vi "StreamDAQ.vi"(1 "Control refDes array":string[][](array[string]), 5 "Control Data Type":dbl[](array[numeric]), 7 "Logging Queue":refnum<queue>, 9 "StreamCluster_TypeDef":T1={"DAQ_Configs"=[], "CTR_Config"={"CTR refDes"="CTR001", "CTR IP Addr"="localhost", "Restart"=FALSE}, "Network_Configs"={"Buffer"=1, "ManagmentRate_Hz"=1000, "StreamRate_Hz"=10, "ConnectionHysterisis"=0, "LoggingRate_Hz"=10}, "ConfigXML_Checksum"=""}, 11 "error in":errorcluster) -> (6 "Control Data Out":dbl[](array[numeric]), 10 "StreamCluster_TypeDef":T1={"DAQ_Configs"=[], "CTR_Config"={"CTR refDes"="CTR001", "CTR IP Addr"="localhost", "Restart"=FALSE}, "Network_Configs"={"Buffer"=1, "ManagmentRate_Hz"=1000, "StreamRate_Hz"=10, "ConnectionHysterisis"=0, "LoggingRate_Hz"=10}, "ConfigXML_Checksum"=""}, 15 "error out":errorcluster)   [LabVIEW 2024]
uses:
  OneDrive - Embry-Riddle Aeronautical University/Admin/Facilities/TC3/TC3 DAC/Code/RTC_PXIe-Code v1_9_0 CODE/QMH-Architecture/support/Control/StreamCluster_TypeDef.ctl
  Control/streamIO_states.ctl
panel:
  out "timed out? 2":bool
  out "timed out?":bool
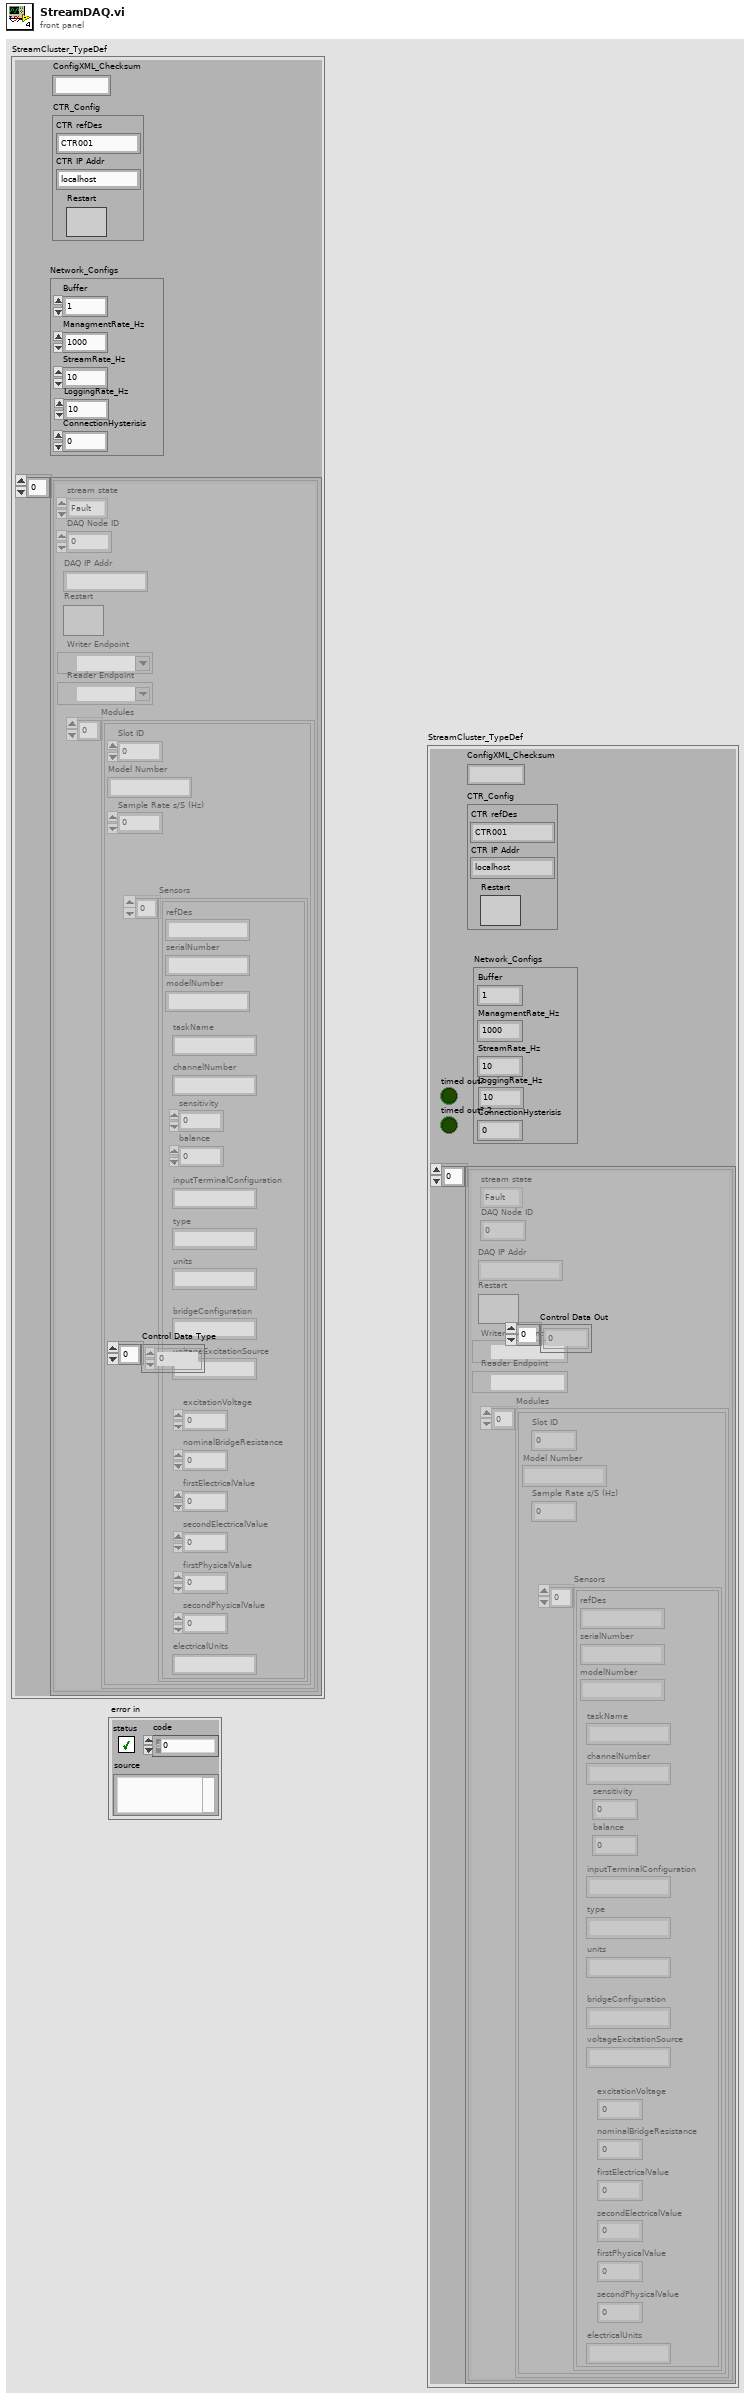
[diagram p1: front panel]
types:
  T1 = typedef "StreamCluster_TypeDef.ctl" = cluster{"DAQ_Configs":cluster{"stream state":T2, "DAQ Node ID":i32, "Writer Endpoint":refnum<k21>, "Reader Endpoint":refnum<k21>, "Modules":cluster{"Slot ID":i32, "Model Number":string, "Sample Rate s/S (Hz)":dbl, "Sensors":cluster{"refDes":string, "serialNumber":string, "modelNumber":string, "units":string, "balance":dbl, "sensitivity":dbl, "type":string, "inputTerminalConfiguration":string, "channelNumber":string, "taskName":string, "bridgeConfiguration":string, "excitationVoltage":dbl, "voltageExcitationSource":string, "nominalBridgeResistance":dbl, "firstElectricalValue":dbl, "secondElectricalValue":dbl, "firstPhysicalValue":dbl, "secondPhysicalValue":dbl, "electricalUnits":string}[]}[], "DAQ IP Addr":string, "Restart":bool}[], "CTR_Config":cluster{"CTR refDes":string, "CTR IP Addr":string, "Restart":bool}, "Network_Configs":cluster{"Buffer":i32, "ManagmentRate_Hz":i32, "StreamRate_Hz":i32, "ConnectionHysterisis":i32, "LoggingRate_Hz":i32}, "ConfigXML_Checksum":string}
  T2 = typedef "streamIO_states.ctl" = enum16{"Fault", "Initialize", "Stream", "Close"}
  T3 = cluster{"stream state":T2, "DAQ Node ID":i32, "Writer Endpoint":refnum<k21>, "Reader Endpoint":refnum<k21>, "Modules":cluster{"Slot ID":i32, "Model Number":string, "Sample Rate s/S (Hz)":dbl, "Sensors":cluster{"refDes":string, "serialNumber":string, "modelNumber":string, "units":string, "balance":dbl, "sensitivity":dbl, "type":string, "inputTerminalConfiguration":string, "channelNumber":string, "taskName":string, "bridgeConfiguration":string, "excitationVoltage":dbl, "voltageExcitationSource":string, "nominalBridgeResistance":dbl, "firstElectricalValue":dbl, "secondElectricalValue":dbl, "firstPhysicalValue":dbl, "secondPhysicalValue":dbl, "electricalUnits":string}[]}[], "DAQ IP Addr":string, "Restart":bool}[]
  T4 = cluster{"stream state":T2, "DAQ Node ID":i32, "Writer Endpoint":refnum<k21>, "Reader Endpoint":refnum<k21>, "Modules":cluster{"Slot ID":i32, "Model Number":string, "Sample Rate s/S (Hz)":dbl, "Sensors":cluster{"refDes":string, "serialNumber":string, "modelNumber":string, "units":string, "balance":dbl, "sensitivity":dbl, "type":string, "inputTerminalConfiguration":string, "channelNumber":string, "taskName":string, "bridgeConfiguration":string, "excitationVoltage":dbl, "voltageExcitationSource":string, "nominalBridgeResistance":dbl, "firstElectricalValue":dbl, "secondElectricalValue":dbl, "firstPhysicalValue":dbl, "secondPhysicalValue":dbl, "electricalUnits":string}[]}[], "DAQ IP Addr":string, "Restart":bool}
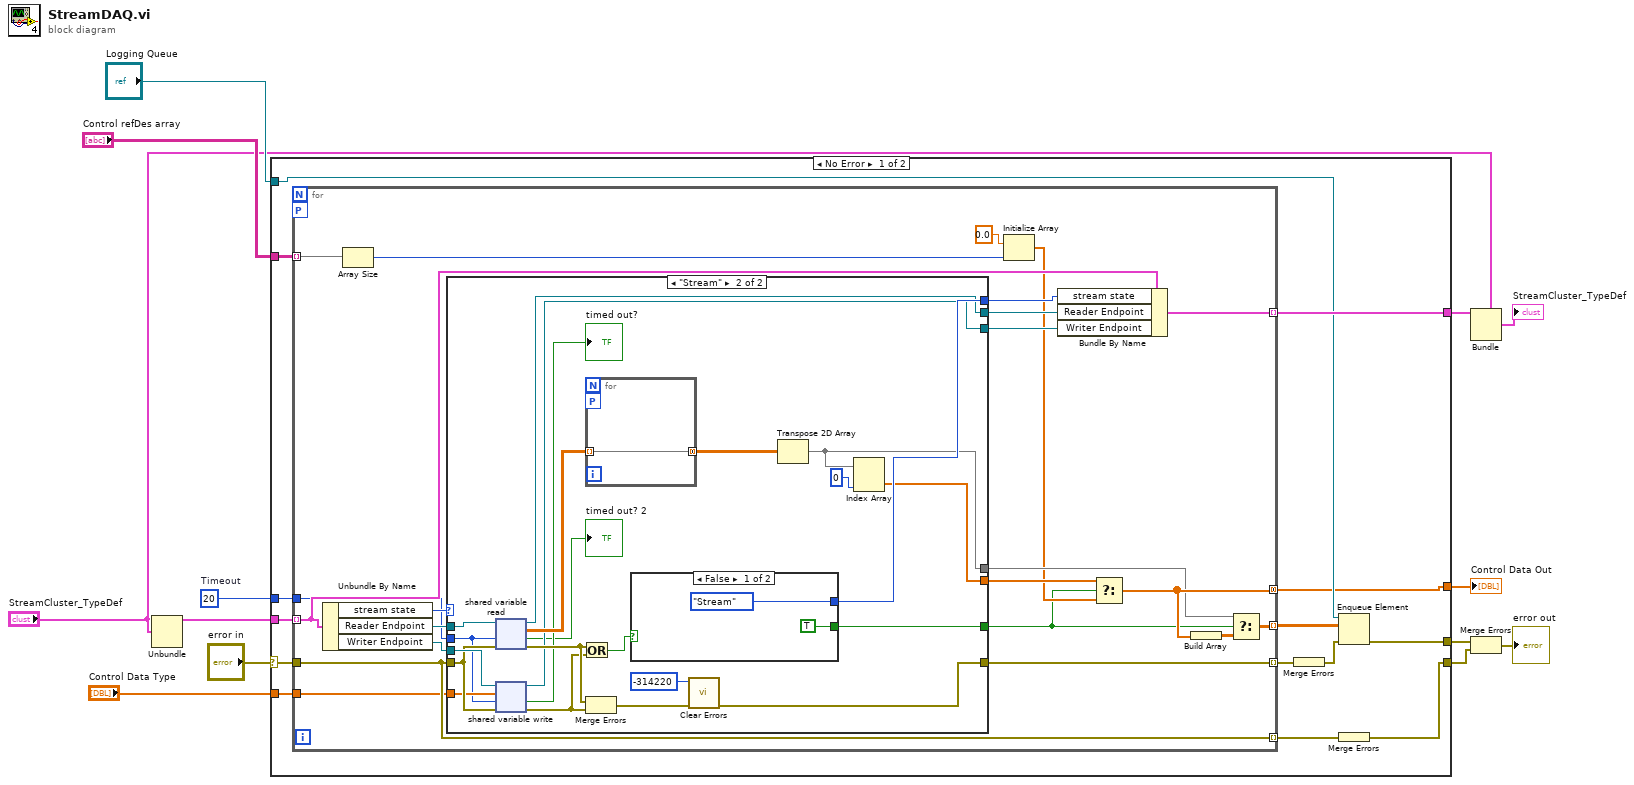
[diagram p0: block diagram]
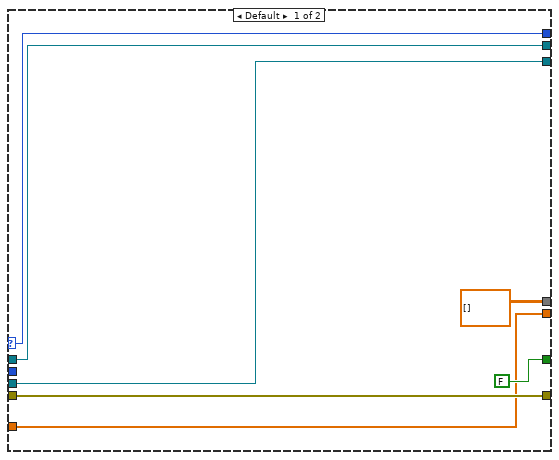
[diagram p2: hidden frame]
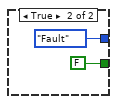
[diagram p3: hidden frame]
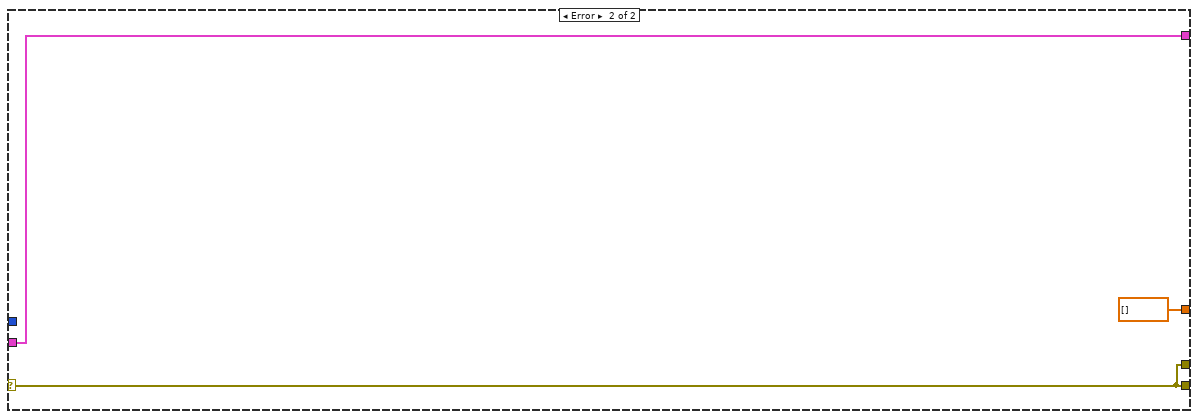
[diagram p4: hidden frame]
diagram:
  w11 = 20  # Timeout
  n1 = Unbundle("StreamCluster_TypeDef") -> ("DAQ_Configs"=w6:T3)  [unwired: 3 out]
  n2 = case shown="No Error" "error in" {
    selector: "error in" -> [w25 w86]
    tunnel: w6 -> [w15 w85]
    tunnel: [w27 w85] -> w4
    tunnel: [w20 w86] -> w13
    tunnel: w11 -> [w26 _]
    tunnel: "Logging Queue" -> [w24 _]
    tunnel: [w21 w86] -> w8
    tunnel: [w17 dbl[] []] -> w1
    tunnel: "Control refDes array" -> [w16 _]
    tunnel: "Control Data Type" -> [w14 _]
    frame No Error {
      n3 = for {
        tunnel: w15 -> [w45] mode=indexing
        tunnel: [w44] -> w27 mode=indexing
        tunnel: [w46] -> w19 mode=indexing
        tunnel: w25 -> [w46]
        tunnel: w26 -> [w40]
        tunnel: [w28] -> w18 mode=indexing
        tunnel: [w39] -> w22 mode=indexing
        tunnel: [w34] -> w17 mode=concatenating
        tunnel: w16 -> [w38] mode=indexing
        workers-P: _ -> [_]
        tunnel: w14 -> [w29]
        n4 = Unbundle By Name(w45) -> ("stream state"=w49:T2, "Reader Endpoint"=w48:refnum<k21>, "Writer Endpoint"=w47:refnum<k21>)
        n5 = Array Size(array=w38) -> (size(s)=w37:i32)
        n6 = case shown="\"Stream\"" w49 {
          selector: w49 -> [w54 _]
          tunnel: w48 -> [w56 w78]
          tunnel: w47 -> [w55 w77]
          tunnel: w46 -> [w53 w76]
          tunnel: [w54 w74] -> w43
          tunnel: [w56 w63] -> w42
          tunnel: [w55 w64] -> w41
          tunnel: w40 -> [_ w62]
          tunnel: [dbl[][] [] w70] -> w32
          tunnel: [w53 w60] -> w39
          tunnel: [w50 w69] -> w33
          tunnel: [FALSE w68] -> w30
          tunnel: w29 -> [w50 w65]
          frame Default {
          }
          frame "Stream" {
            n7 = shared-variable-read(w78, w76, w62) -> (w63:refnum<k21>, w67:errorcluster, →"timed out? 2":bool, w73:dbl[][][])  [unwired: 1 in]
            n8 = shared-variable-write(w77, w76, w65, w62) -> (w64:refnum<k21>, w66:errorcluster, →"timed out?":bool)
            n9 = Or(x=w67, y=w66) -> (x .or. y?=w75:bool)
            n10 = for {
              tunnel: w73 -> [w79] mode=indexing
              tunnel: [w79] -> w72 mode=concatenating
              workers-P: _ -> [_]
            }
            n11 = Merge Errors(w67, w66) -> (w61:errorcluster)
            n12 = case shown="False" w75 {
              tunnel: [streamIO_states."Stream" ("stream state") streamIO_states."Fault" ("stream state")] -> w74
              tunnel: [TRUE FALSE] -> w68
              frame False {
              }
              frame True {
              }
            }
            n13 = call <vilib>:"Clear Errors.vi"("error in (no error)"=w61, "specific error code to clear (0: all)"=-314220) -> ("error out"=w60:errorcluster)  [unwired: 4 in, 1 out]
            n14 = Transpose 2D Array(2D array=w72) -> (transposed array=w70:dbl[][])
            n15 = Index Array(array=w70, index (col)=0) -> (element=w69:dbl[])  [unwired: 1 in]
          }
        }
        n16 = Initialize Array(0.0 ("element"), w37) -> (w31:dbl[])
        n17 = Bundle By Name(cluster=w45, "stream state"=w43, "Reader Endpoint"=w42, "Writer Endpoint"=w41) -> (w44:T4)
        n18 = Select(t=w33, s=w30, f=w31) -> (s? t:f=w34:dbl[])
        n19 = Build Array(w34) -> (w35:dbl[][])
        n20 = Select(t=w32, s=w30, f=w35) -> (s? t:f=w28:dbl[][])
      }
      n21 = Merge Errors(w22) -> (w23:errorcluster)
      n22 = Enqueue Element(queue=w24, element=w18, error in (no error)=w23) -> (error out=w21:errorcluster)  [unwired: 1 in, 2 out]
      n23 = Merge Errors(w19) -> (w20:errorcluster)
    }
    frame Error {
    }
  }
  "Control Data Out" <- w1
  n24 = Bundle(cluster="StreamCluster_TypeDef", "DAQ_Configs"=w4) -> (→"StreamCluster_TypeDef":T1)  [unwired: 3 in]
  n25 = Merge Errors(w8, w13) -> (→"error out":errorcluster)
